vi "phi_offset.vi"(8 "error in":errorcluster, 9 "yaw":dbl, 10 "roll":dbl, 11 "pitch":dbl) -> (0 "error out":errorcluster, 2 "phi":dbl)   [LabVIEW 2011, in "gVision.lvlib"]
uses:
  gVision.lvlib
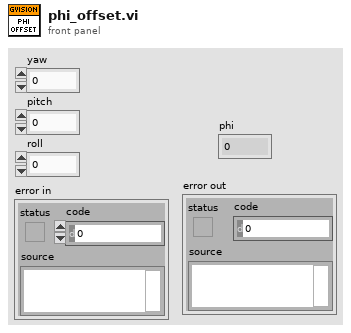
[diagram p1: front panel]
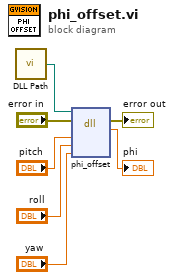
[diagram p0: block diagram]
diagram:
  n1 = call "DLL Path.vi"() -> ("DLL Path"=w7:path)  [unwired: 5 in]
  n2 = dll-call lib="?" fn="phi_offset"(path in=w7, error in="error in", "pitch"="pitch", "roll"="roll", "yaw"="yaw") -> (error out=→"error out":errorcluster, "phi"=→"phi":dbl)  [unwired: 4 in, 1 out]
